vi "BASE.Create.vi"(8 "error in (no error)":errorcluster, 11 "BASE in":refnum<class "BASE.lvclass">) -> (0 "error out":errorcluster, 3 "BASE out":refnum<class "BASE.lvclass">)   [LabVIEW 2019, in "BASE.lvlib" / "BASE.lvclass"]
uses:
  BASE.lvclass
  BASE.lvclass/BASE.ctl
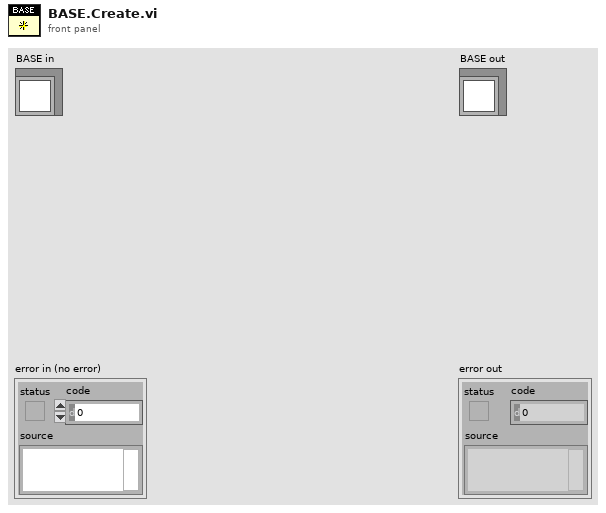
[diagram p1: front panel]
types:
  T1 = typedef "BASE.lvlib/BASE.lvclass/privateData--reference.ctl" = refnum<data-value>
  T2 = typedef "BASE.lvlib/BASE.lvclass/privateData--cluster.ctl" = cluster{"Config":T3, "Configured?":bool}
  T3 = typedef "BASE.lvlib/BASE.lvclass/config--cluster.ctl" = cluster{"Config Path":path}
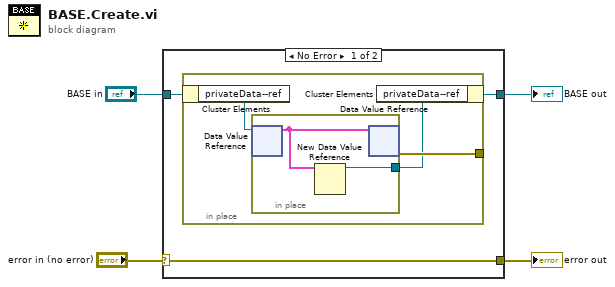
[diagram p0: block diagram]
diagram:
  n1 = case shown="No Error" "error in (no error)" {
    selector: "error in (no error)" -> [w5 w13]
    tunnel: "BASE in" -> [w7 w14]
    tunnel: [w6 w14] -> w1
    tunnel: [w5 w13] -> w2
    frame No Error {
      n2 = in-place {
        in-place-border: [w9] -> _
        n3 = in-place-cluster #1(w7) -> ("privateData--ref"=w10:T1)
        n4 = in-place {
          in-place-border: [w12] -> w8
          n5 = in-place-dvr #2(w10) -> (w11:T2)  [unwired: 1 out]
          n6 = New Data Value Reference(data value=w11) -> (data value reference=w12:refnum<data-value>)  [unwired: 1 in, 1 out]
          n7 = in-place-dvr #2(w11) -> (w9:errorcluster)  [unwired: 1 out]
        }
        n8 = in-place-cluster #1("privateData--ref"=w8) -> (w6:refnum<class "BASE.lvclass">)
      }
    }
    frame Error {
    }
  }
  "error out" <- w2
  "BASE out" <- w1
